vi "File_Application  Path INI Location.vi"(1 "Name of System (Save as Default)":string="MySystem.ini") -> (0 "Path INI Location":path)   [LabVIEW 2020]
uses:
  <vilib>/Utility/sysdir.llb/System Directory Type.ctl
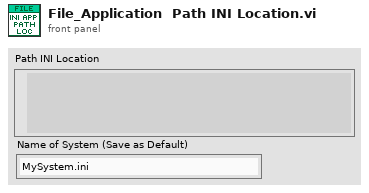
[diagram p1: front panel]
types:
  T1 = typedef "System Directory Type.ctl" = i32
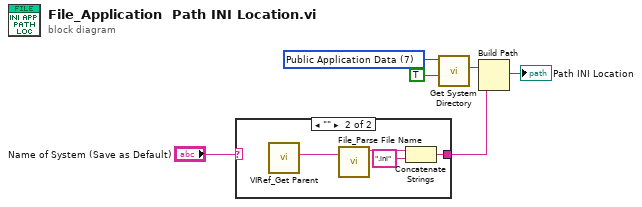
[diagram p0: block diagram]
diagram:
  w3 = T1 7 items=["User Home"=0, "User Desktop"=1, "User Documents"=2, "User Application Data"=3, "User Preferences"=4, "User Temporary"=5, "Public Documents"=6, "Public Application Data"=7, "Public Preferences"=8, "Public Cache"=13, "System Core Libraries"=9, "System Installed Libraries"=10, "Application Files"=11, "Boot Volume Root"=12] ("system directory type")
  n1 = case shown="\"\"" "Name of System (Save as Default)" {
    selector: "Name of System (Save as Default)" -> [w7 _]
    tunnel: [w7 w8] -> w2
    frame "False", Default {
    }
    frame "" {
      n2 = call "VIRef_Get Parent.vi"() -> ("Parent Vi Name Out"=w11:string)  [unwired: 8 in, 3 out]
      n3 = call "File_Parse File Name.vi"("File Name"=w11) -> ("File Name Out"=w10:string)  [unwired: 4 in, 2 out]
      n4 = Concatenate Strings(w10, ".ini" ("string")) -> (w8:string)
    }
  }
  n5 = call <vilib>:"Get System Directory.vi"("create directory if not found? (F)"=TRUE, "system directory type"=w3) -> ("system directory"=w5:path)  [unwired: 9 in]
  n6 = Build Path(base path=w5, name or relative path=w2) -> (appended path=→"Path INI Location":path)
